vi "Send Get N Images.vi"(6 "timeout in ms (-1)":i32=-1, 7 "Message Priority (Normal)":T1=enum."Normal", 8 "error in":errorcluster, 10 "count (-1 = all)":i32=-1, 11 "Message Enqueuer":refnum<class "Message Enqueuer.lvclass">) -> (0 "error out":errorcluster, 1 "timed out?":bool, 2 "Reply":refnum<class "Generic Image.lvclass">[](array[class]), 3 "Message Enqueuer out":refnum<class "Message Enqueuer.lvclass">)   [LabVIEW 2024, in "Camera Worker.lvlib" / "Get N Images Msg.lvclass"]
doc: "This VI sends the message to an actor."
uses:
  Get N Images Msg.lvclass
  Get N Images Msg.lvclass/Get N Images Msg.ctl
  Camera Worker/Reply Msg Generic Image Arr/Reply Msg Generic Image Arr.lvclass
  <vilib>/ActorFramework/Message Enqueuer/Message Enqueuer.lvclass
  <vilib>/ActorFramework/Message Enqueuer/Message Priority.ctl
  Typedefs/Generic Image/Generic Image.lvclass
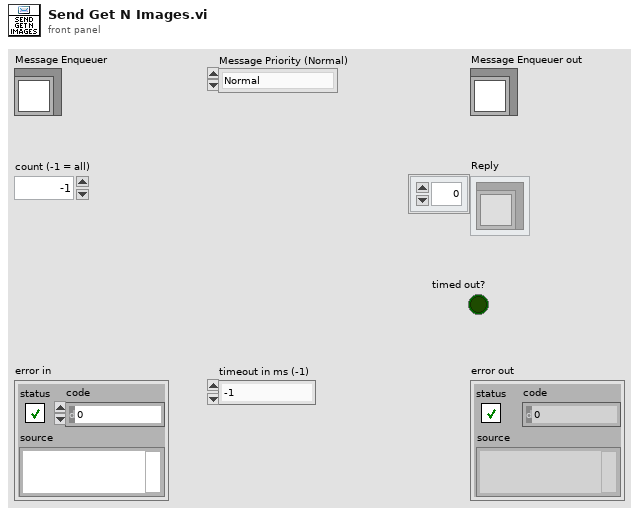
[diagram p1: front panel]
types:
  T1 = typedef "Actor Framework.lvlib/Message Enqueuer.lvclass/Message Priority.ctl" = enum16{"Low", "Normal", "High"}
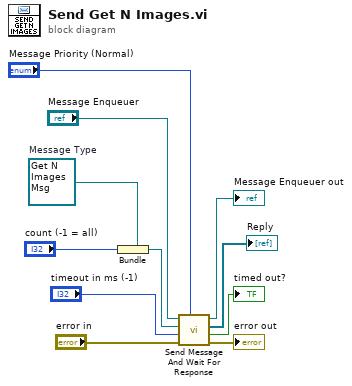
[diagram p0: block diagram]
diagram:
  w6 = refnum<class "Get N Images Msg.lvclass"> refnum  # Message Type
  n1 = Bundle(cluster=w6, "count (-1 = all)") -> (w3:refnum<class "Get N Images Msg.lvclass">)
  n2 = call "Send Message And Wait For Response.vi"("Message Priority (Normal)"="Message Priority (Normal)", "error in (no error)"="error in", "timeout in ms (-1)"="timeout in ms (-1)", "Original Message"=w3, "Message Enqueuer in"="Message Enqueuer") -> ("error out"=→"error out":errorcluster, "timed out?"=→"timed out?":bool, "Reply"=→"Reply":refnum<class "Generic Image.lvclass">[], "Message Enqueuer out"=→"Message Enqueuer out":refnum<class "Message Enqueuer.lvclass">)  [unwired: 3 in]
